vi "niFpgaPID_Wrapper.vi"   [LabVIEW 2017]
doc: "Implements a single-precision floating-point PID algorithm for PID applications with high-speed control and/or high channel count on an FPGA target. You can use this VI to create single-channel, multi-channel, and multi-rate control applications."
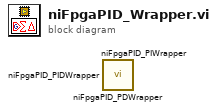
[diagram p0: block diagram]
diagram:
  n1 = call <vilib>:"niFpgaPID_PDWrapper.vi"() -> ()  [unwired: 13 in, 3 out]
  n2 = call <vilib>:"niFpgaPID_PIWrapper.vi"() -> ()  [unwired: 13 in, 3 out]
  n3 = call <vilib>:"niFpgaPID_PIDWrapper.vi"() -> ()  [unwired: 13 in, 3 out]
